vi "SeparateValueAndUnit.vi"(11 "input value string":string) -> (2 "unit":string, 3 "value":dbl)   [LabVIEW 2018, in "Library-DataConvert.lvlib"]
uses:
  Library-DataConvert.lvlib
  <vilib>/regexp/Match Regular Expression.xnode
  <vilib>/Utility/error.llb/whitespace.ctl
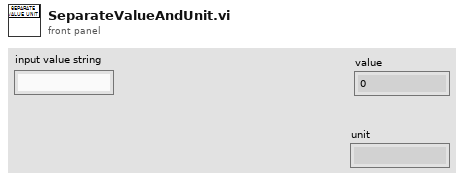
[diagram p1: front panel]
types:
  T1 = typedef "whitespace.ctl" = u16
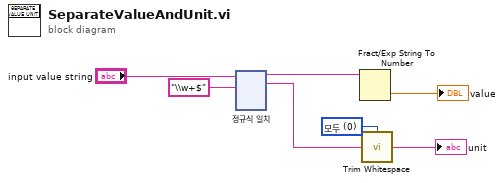
[diagram p0: block diagram]
diagram:
  w5 = T1 0 items=["모두", "문자열의 시작", "문자열의 끝"] ("location (both)")
  n1 = xnode "정규식 일치"("입력 문자열"="input value string", "정규식"="\\w+$") -> ("일치 구문 앞"=w2:string, "전체 일치 구문"=w1:string)  [unwired: 4 in, 3 out]
  n2 = Fract/Exp String To Number(string=w2) -> (number=→"value":dbl)  [unwired: 3 in, 1 out]
  n3 = call <vilib>:"Trim Whitespace.vi"("string"=w1, "location (both)"=w5) -> ("trimmed string"=→"unit":string)
